vi "projet.vi"() -> (0 "Bon cannette":dbl, 1 "Numeric":i32)   [LabVIEW 2023]
uses:
  Control 1.ctl
  Control 5.ctl
  <vilib>/numeric/Random Number (Range) U64.vi
  <vilib>/numeric/sub_Random U32.vi
panel:
  in  "OK Button 3":bool
  out "MP3 2":bool
  out "Valeur PH":dbl
  out "Boolean":bool
  in  "Seuil PH":dbl(slide) scale=0.0..14.0
  in  "stop":bool
  out "Tab Control":T1(tab)
  in  "StartB":bool
  in  "Radio Buttons":enum32{"Radio Selection 1", "Radio Selection 2"}(radio)
  in  "?":bool
  in  "Cancel Button":bool
  in  "OK Button":bool
  in  "Cancel Button 2":bool
  in  "OK Button 2":bool
  out "MP3":bool
  out "Tank":cluster{dbl, dbl}(slide)={0.0, 10.0} scale=0.0..10.0
  # "DO u want gaz ?"
  # "DO u want sugar ?"
  # "Production finie"
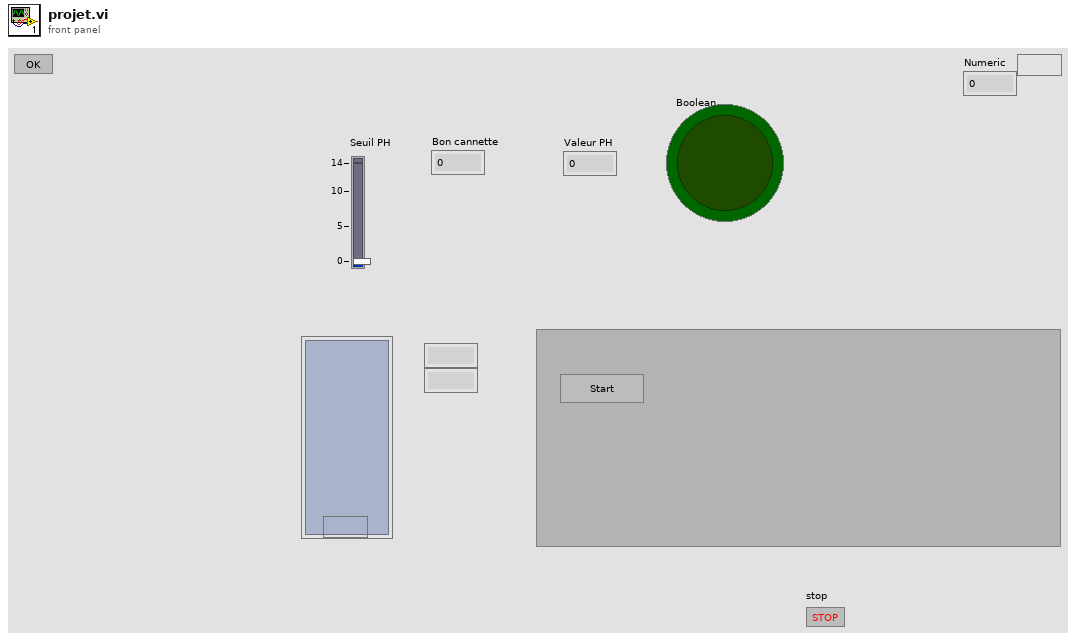
[diagram p1: front panel]
types:
  T1 = enum32{"Start", "Type", "preparer", "GazS", "GazF", "Sugar", "Finish"}
  T2 = typedef "Control 1.ctl" = enum32{"Start", "Page 1", "Page 2", "Page 3", "Page 4", "Sugar", "Finish"}
  T3 = typedef "Control 5.ctl" = enum32{"Start", "Page 1", "Page 2", "Page 3", "Page4"}
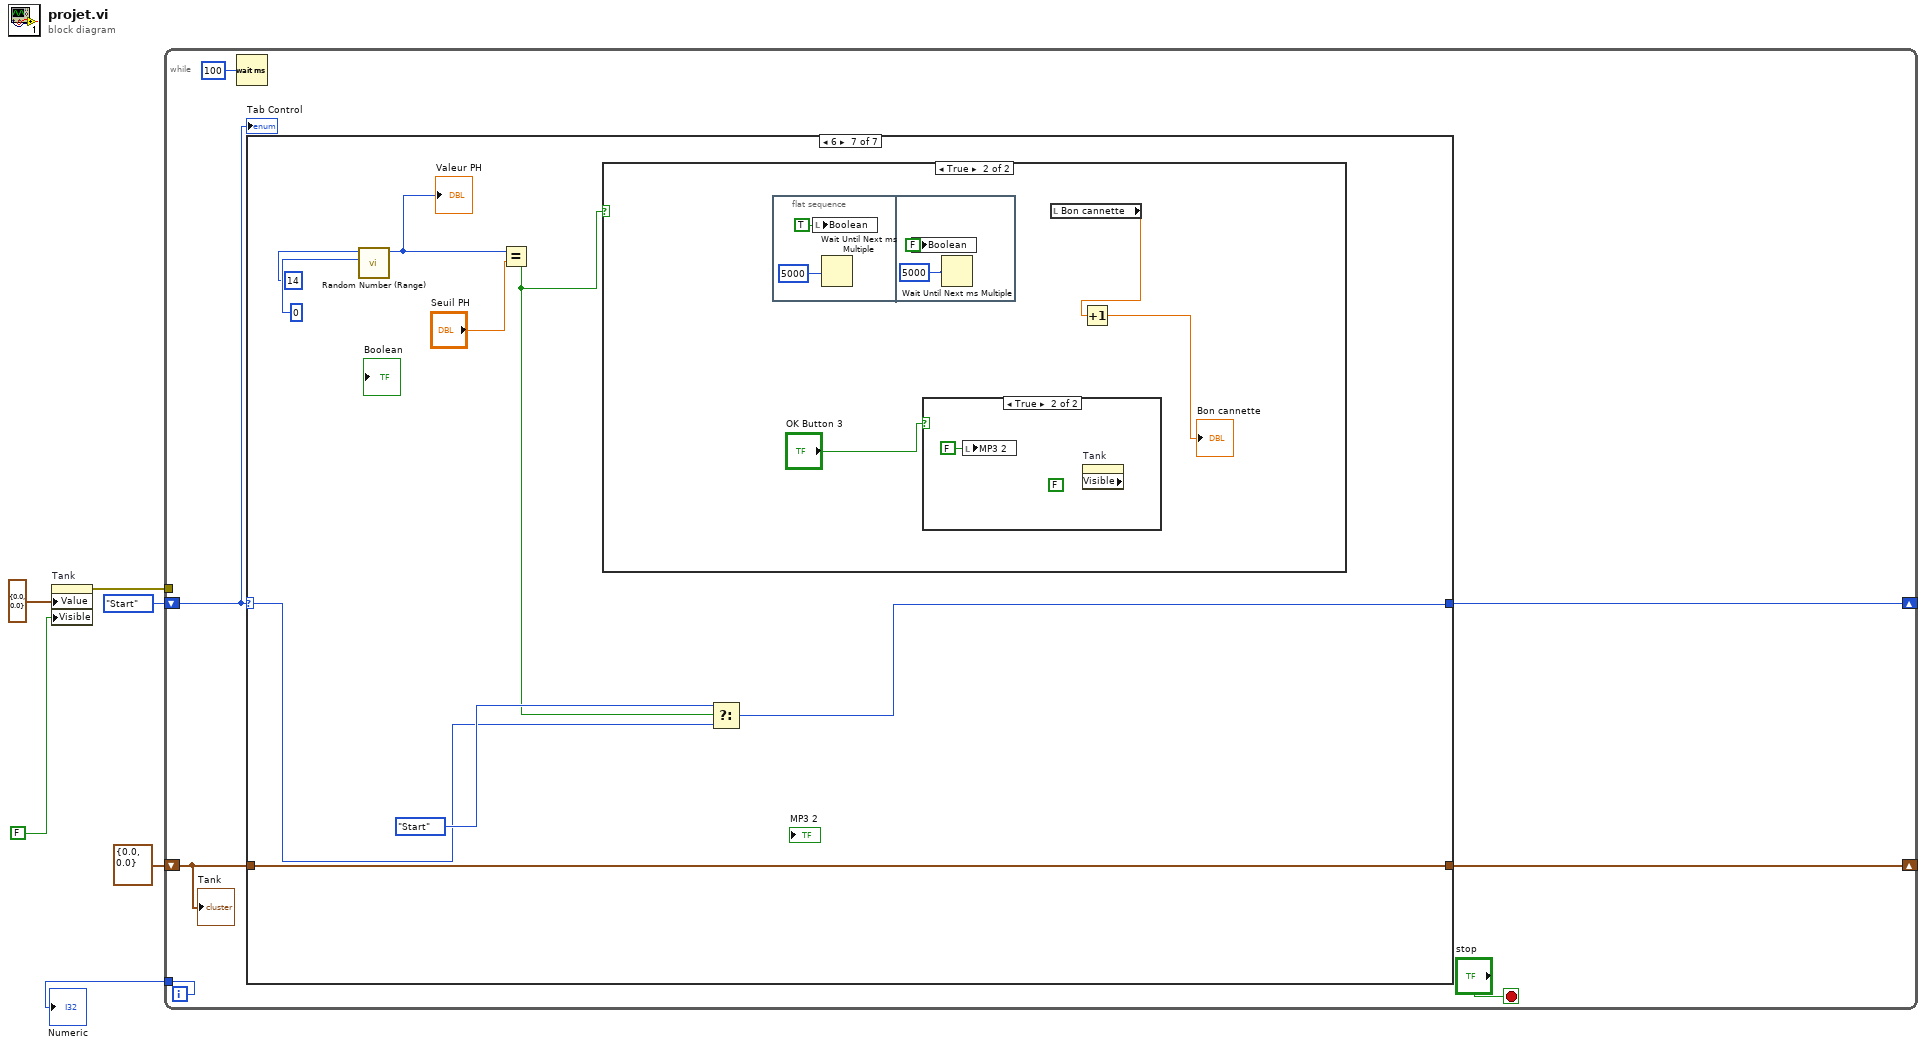
[diagram p0: block diagram]
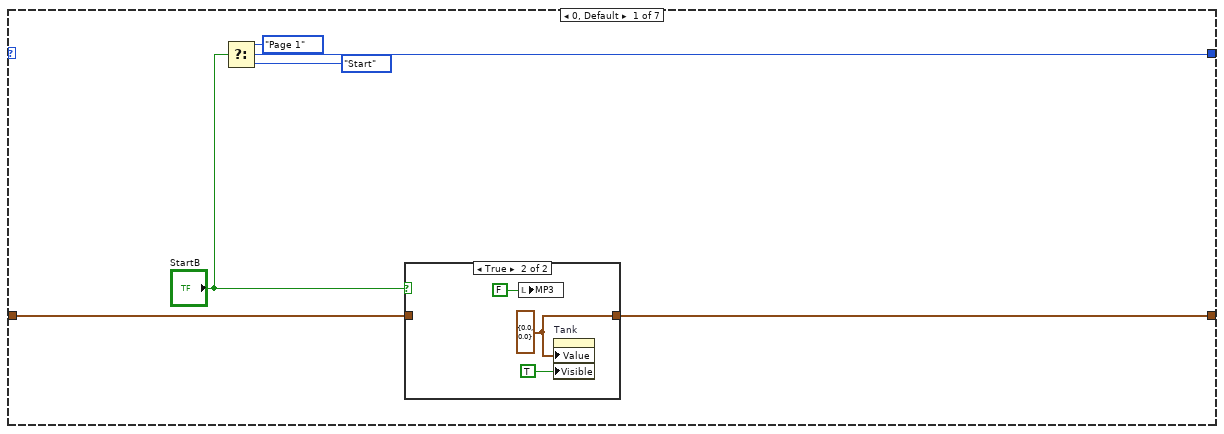
[diagram p2: hidden frame]
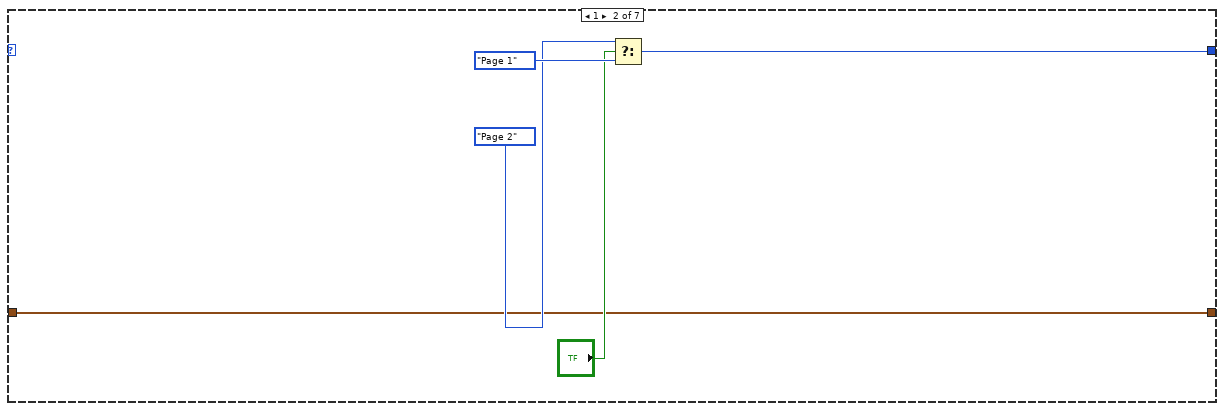
[diagram p4: hidden frame]
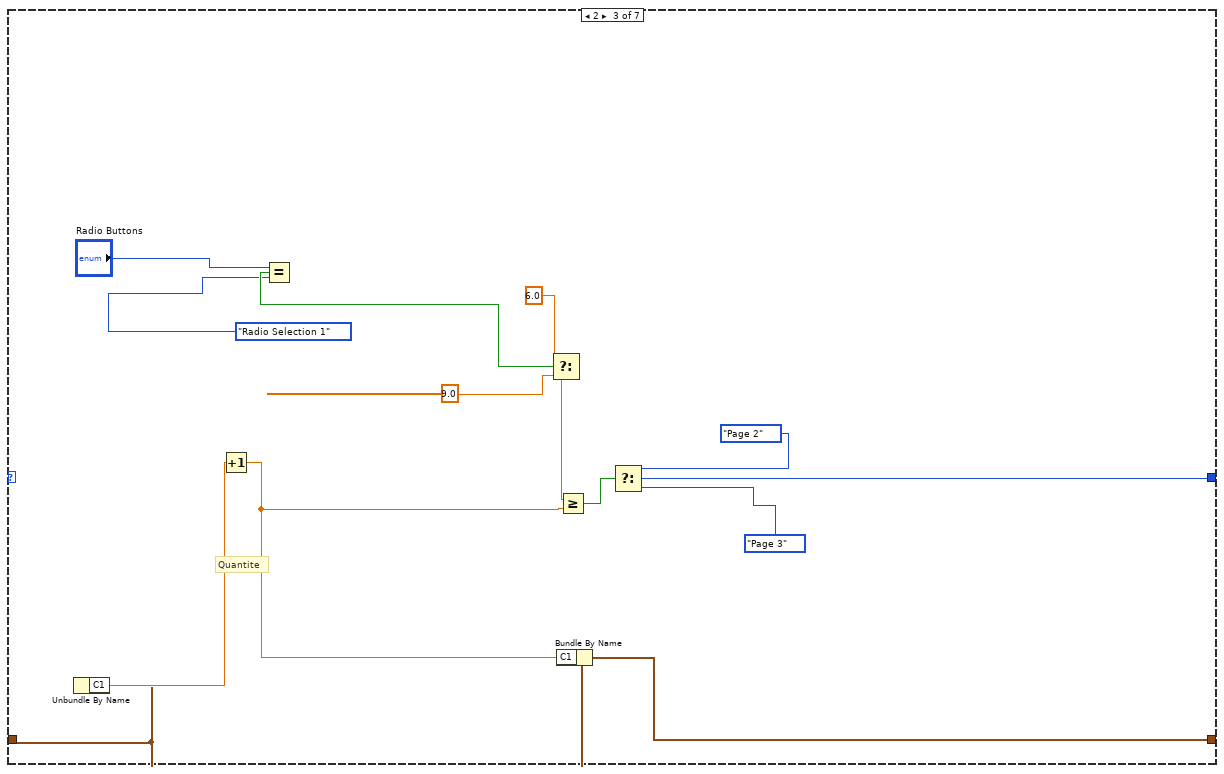
[diagram p5: hidden frame]
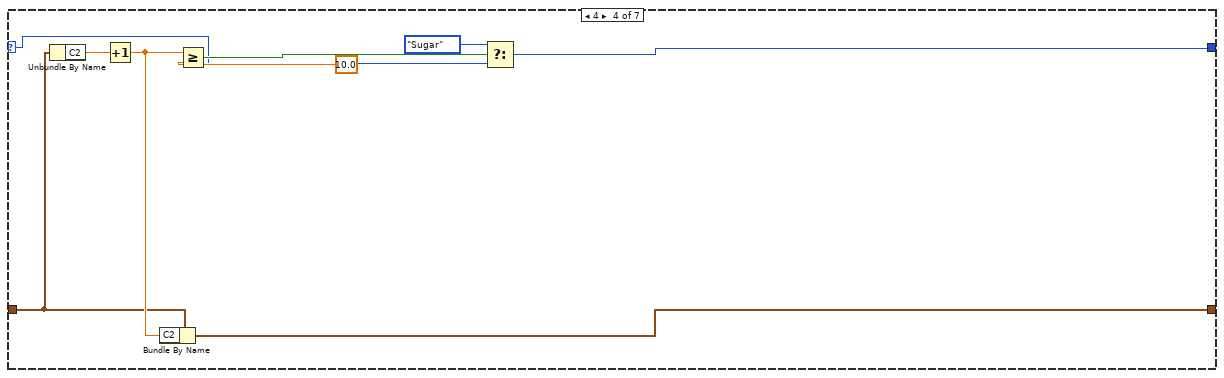
[diagram p6: hidden frame]
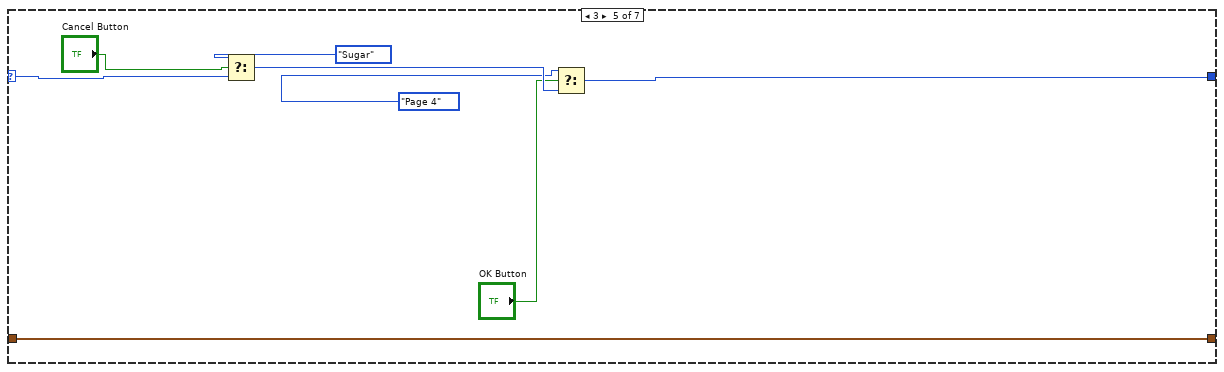
[diagram p7: hidden frame]
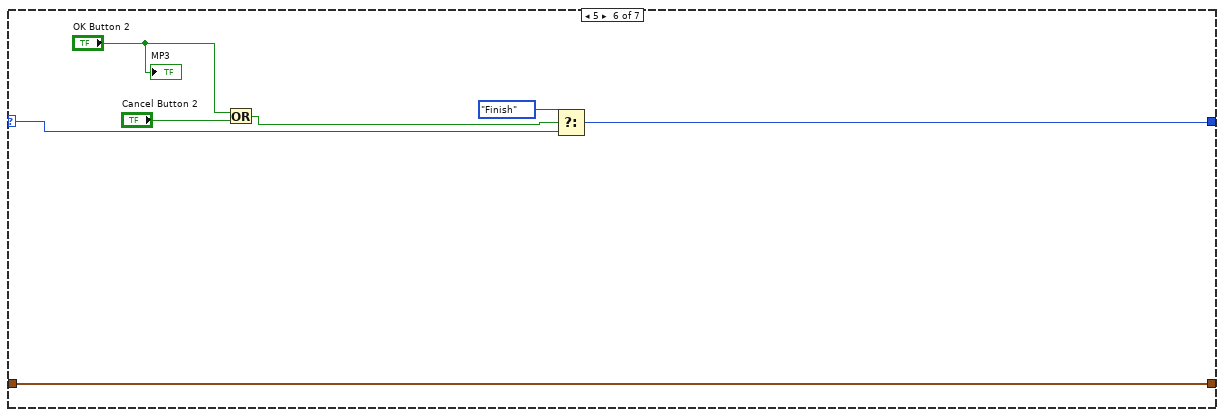
[diagram p8: hidden frame]
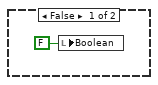
[diagram p9: hidden frame]
diagram:
  n1 = property on="Tank" class="Slide (strict)"("Value"=cluster{dbl, dbl} {0.0, 0.0} ("Tank"), "Visible"=FALSE) -> (error out=w3:errorcluster)  [unwired: 2 in, 1 out]
  n2 = while {
    shift-right: [w12] -> _
    shift-left: cluster{"C1":dbl, "C2":dbl} {"C1"=0.0, "C2"=0.0} ("Tank") -> [w9]
    shift-right: [w10] -> _
    shift-left: Control_1."Start" ("Tab Control") -> [w11]
    tunnel: w3 -> [_]
    tunnel: [w7] -> w1
    i -> [w7]
    stop <- "stop" stop-if-true
    n3 = Wait (ms)(milliseconds to wait=u32 100 ("millisecond timer value")) -> ()  [unwired: 1 out]
    n4 = case shown="6" w11 {
      selector: w11 -> [_ _ _ w45 w58 w64 w73]
      tunnel: [w16 w25 w31 w43 w55 w61 w72] -> w10
      tunnel: w9 -> [w15 w24 w36 w47 w52 w66 w75]
      tunnel: [w14 w24 w35 w46 w52 w66 w75] -> w12
      frame 0, Default {
        n5 = Select(t=Control_5."Page 1" ("Tab Control"), s="StartB", f=Control_5."Start" ("Tab Control")) -> (s? t:f=w16:T3)
        n6 = case shown="True" "StartB" {
          tunnel: [w20 w21] -> w14
          tunnel: w15 -> [w20 _]
          frame False {
          }
          frame True {
            w21 = cluster{dbl, dbl} {0.0, 0.0} ("Tank")
            n7 = local write "MP3"(FALSE ("MP3")) -> ()
            n8 = property on="Tank" class="Slide (strict)"("Value"=w21, "Visible"=TRUE) -> ()  [unwired: 2 in, 2 out]
          }
        }
      }
      frame 1 {
        n9 = Select(t=Control_5."Page 2" ("Tab Control"), s="?", f=Control_5."Page 1" ("Tab Control")) -> (s? t:f=w25:T3)
      }
      frame 2 {
        # "Quantite"
        n10 = Unbundle By Name(w36) -> ("C1"=w37:dbl)
        n11 = Increment(x=w37) -> (x+1=w30:dbl)
        n12 = Equal?(x="Radio Buttons", y=enum32{"Radio Selection 1", "Radio Selection 2"}."Radio Selection 1" ("x")) -> (x = y?=w40:bool)
        n13 = Select(t=6.0, s=w40, f=9.0) -> (s? t:f=w29:dbl)
        n14 = Bundle By Name(cluster=w36, "C1"=w30) -> (w35:cluster{"C1":dbl, "C2":dbl})
        n15 = Greater Or Equal?(x=w29, y=w30) -> (x >= y?=w32:bool)
        n16 = Select(t=Control_5."Page 2" ("Tab Control"), s=w32, f=Control_5."Page 3" ("Tab Control")) -> (s? t:f=w31:T3)
      }
      frame 4 {
        n17 = Unbundle By Name(w47) -> ("C2"=w51:dbl)
        n18 = Increment(x=w51) -> (x+1=w50:dbl)
        n19 = Bundle By Name(cluster=w47, "C2"=w50) -> (w46:cluster{"C1":dbl, "C2":dbl})
        n20 = Greater Or Equal?(x=w50, y=10.0) -> (x >= y?=w49:bool)
        n21 = Select(t=Control_1."Sugar" ("Tab Control"), s=w49, f=w45) -> (s? t:f=w43:u32)
      }
      frame 3 {
        n22 = Select(t=Control_1."Sugar" ("Tab Control"), s="Cancel Button", f=w58) -> (s? t:f=w57:u32)
        n23 = Select(t=Control_1."Page 4" ("Tab Control"), s="OK Button", f=w57) -> (s? t:f=w55:u32)
      }
      frame 5 {
        n24 = Or(x="OK Button 2", y="Cancel Button 2") -> (x .or. y?=w63:bool)
        n25 = Select(t=Control_1."Finish" ("Tab Control"), s=w63, f=w64) -> (s? t:f=w61:u32)
        "MP3" <- "OK Button 2"
      }
      frame 6 {
        n26 = call-poly <vilib>:"Random Number (Range).vi"("lower bound (0)"=u64 0, "upper bound (100)"=u64 14) -> ("number"=w71:u64)  [unwired: 9 in]
        "Valeur PH" <- w71
        n27 = Equal?(x=w71, y="Seuil PH") -> (x = y?=w67:bool)
        n28 = case shown="True" w67 {
          frame False {
            n29 = local write "Boolean"(FALSE ("Boolean")) -> ()
          }
          frame True {
            n30 = flat-sequence {
              frame #0 {
                n31 = local write "Boolean"(TRUE ("Boolean")) -> ()
                n32 = Wait Until Next ms Multiple(millisecond multiple=u32 5000 ("millisecond timer value")) -> ()  [unwired: 1 out]
              }
              frame #1 {
                n33 = local write "Boolean"(FALSE ("Boolean")) -> ()
                n34 = Wait Until Next ms Multiple(millisecond multiple=u32 5000 ("millisecond timer value")) -> ()  [unwired: 1 out]
              }
            }
            n35 = case shown="True" "OK Button 3" {
              frame False {
              }
              frame True {
                (unwired) FALSE ("Visible")
                n36 = local write "MP3 2"(FALSE ("MP3")) -> ()
                n37 = property on="Tank" class="Slide (strict)" props=["Visible"]() -> ()  [unwired: 2 in, 3 out]
              }
            }
            n38 = local read "Bon cannette"() -> (w79:dbl)
            n39 = Increment(x=w79) -> (x+1=→"Bon cannette":dbl)
          }
        }
        n40 = Select(t=Control_1."Start" ("Tab Control"), s=w67, f=w73) -> (s? t:f=w72:u32)
      }
    }
    "Tab Control" <- w11
    "Tank" <- w9
  }
  "Numeric" <- w1
